vi "testVI.vi"(10 "Data in":sgl format="%#_13g") -> ()   [LabVIEW 2015]
uses:
  C:/Users/Arkadiusz/SkyDrive/Dokumenty/Visual Studio 2015/Projects/NordicDatabaseDLL/NordicDatabaseDLL/bin/Debug/NordicDatabaseDLL.dll
  Visual Studio 2015/Projects/NordicDatabaseDLL/NordicDatabaseDLL/bin/Debug/NordicDatabaseDLL.dll
  DBEnum.ctl
panel:
  in  "stop":bool
  in  "OK Button":bool
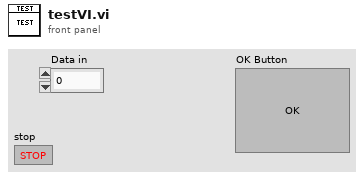
[diagram p1: front panel]
types:
  T1 = typedef "DBEnum.ctl" = enum16{"Temperature", "HeartRate", "XAccelero", "YAccelero", "ZAccelero"}
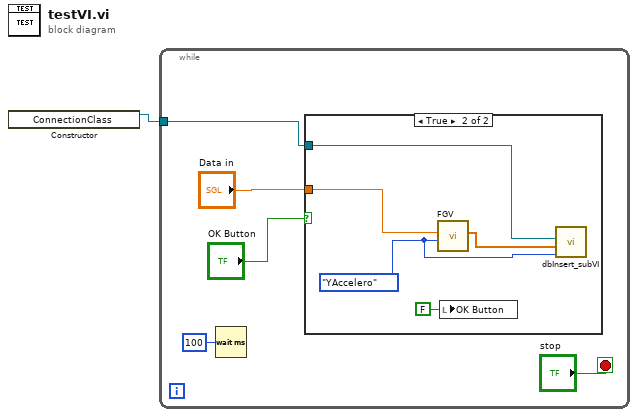
[diagram p0: block diagram]
diagram:
  n1 = constructor class="ConnectionClass"() -> (reference out=w1:refnum<k24>)  [unwired: 3 in, 2 out]
  n2 = while {
    tunnel: w1 -> [w5]
    stop <- "stop" stop-if-true
    n3 = Wait (ms)(milliseconds to wait=u32 100) -> ()  [unwired: 1 out]
    n4 = case shown="True" "OK Button" {
      tunnel: "Data in" -> [_ w11]
      tunnel: w5 -> [_ w8]
      frame False {
      }
      frame True {
        w9 = DBEnum."YAccelero" ("Enum")
        n5 = call "FGV.vi"("Enum"=w9, "Data in"=w11) -> ("Output Array"=w10:sgl[])  [unwired: 9 in]
        n6 = local write "OK Button"(FALSE ("OK Button")) -> ()
        n7 = call "dbInsert_subVI.vi"("Enum"=w9, "Array"=w10, "reference"=w8) -> ()  [unwired: 9 in]
      }
    }
  }
